vi "Stop Core.vi"(10 "final error code":i32, 11 "PVClient-Example in":refnum<class "PVClient-Example.lvclass">) -> (3 "PVClient-Example out":refnum<class "PVClient-Example.lvclass">)   [LabVIEW 2013, in "PVClient-Example.lvlib" / "PVClient-Example.lvclass"]
doc: "(<B>Filename</B>: Actor Framework.lvlib:Actor.lvclass:Stop Core.vi)\n\nDefines what the actor does before it stops. Use the <B>final error code</B> input to determine whether the actor shut down in response to an error.\n\nBy default, this method does nothing. A descendant class may override it to define behavior, such as shutting down any processes the actor initiated in its override of the Actor Core method."
uses:
  PVClient-Example.lvclass
  Core/Actors/CS++BaseActor/CS++BaseActor.lvclass
  PVClient-Example.lvclass/PVClient-Example.ctl
  <vilib>/ActorFramework/Message Enqueuer/Message Enqueuer.lvclass/Message Enqueuer.ctl
  <vilib>/ActorFramework/Message Enqueuer/Enqueue.vi
  <vilib>/ActorFramework/Message Priority Queue/Priority Enqueue.vi
  <vilib>/ActorFramework/Stop Msg/Stop Msg.lvclass
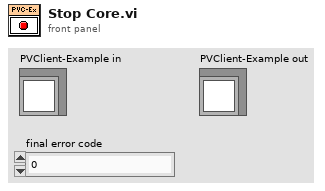
[diagram p1: front panel]
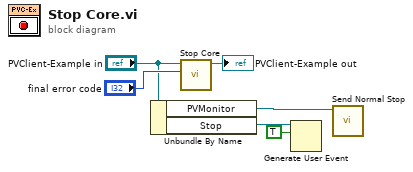
[diagram p0: block diagram]
diagram:
  n1 = Unbundle By Name("PVClient-Example in") -> ("PVMonitor"=w3:refnum<class "Message Enqueuer.lvclass">, "Stop"=w2:refnum<user-event>)
  n2 = call-parent "Stop Core.vi"("final error code"="final error code", "CS++BaseActor in"="PVClient-Example in") -> ("CS++BaseActor out"=→"PVClient-Example out":refnum<class "PVClient-Example.lvclass">)  [unwired: 9 in]
  n3 = Generate User Event(user event=w2, event data cluster=TRUE ("event data")) -> ()  [unwired: 2 in, 2 out]
  n4 = call <vilib>:"Send Normal Stop.vi"("Message Enqueuer"=w3) -> ()  [unwired: 10 in, 1 out]
